vi "inclinometerSerialTest.vi"() -> ()   [LabVIEW 2016]
uses:
  <vilib>/Instr/_visa.llb/VISA Configure Serial Port (Instr).vi
  Common_RT_Modbus/CRC/CRC.lvclass
panel:
  out "result":i32
  out "Response":u8[](array[numeric])
  in  "Command":u8[](array[numeric])=[127, 0, 0, 0, 0, 0, 0, 0, 2, 206, 21] format="%02x"
  in  "SendMany":bool
  out "Time (us)":u32
  in  "Send":bool
  in  "Stop":bool
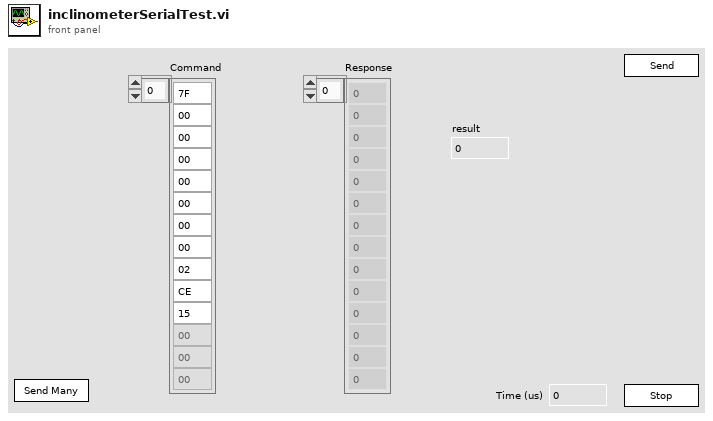
[diagram p1: front panel]
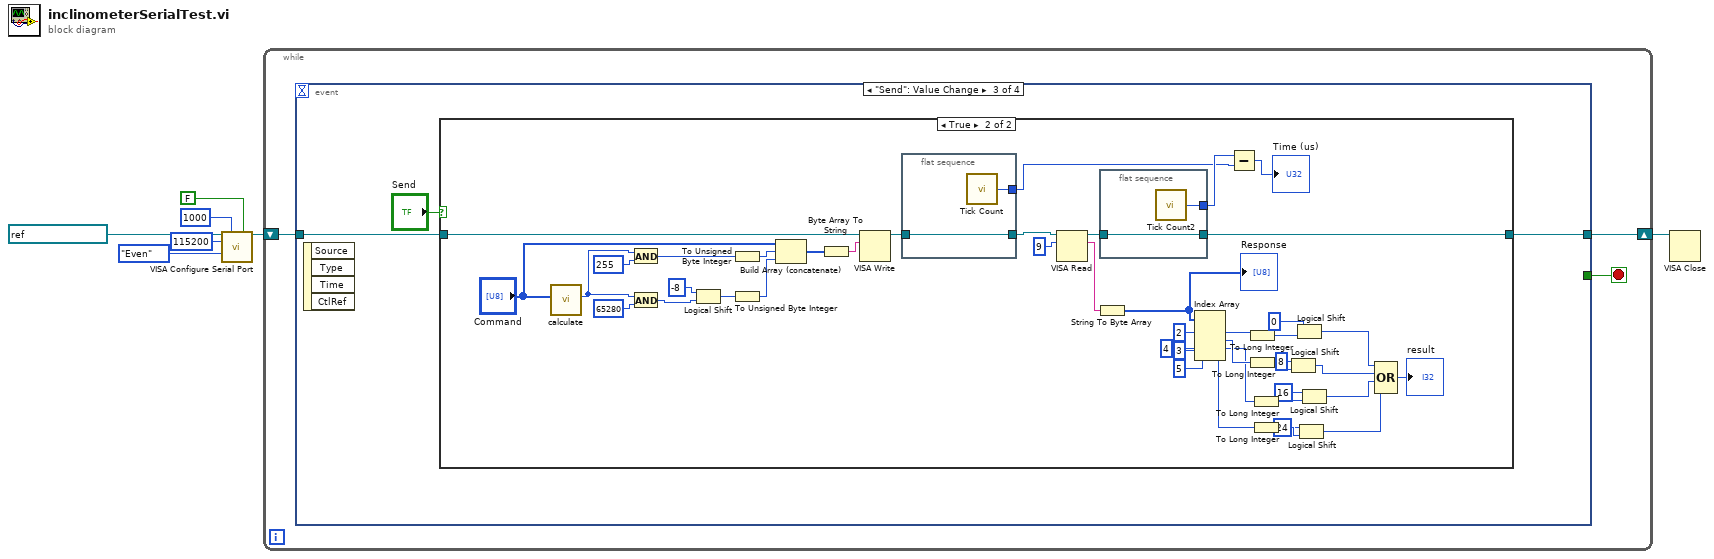
[diagram p0: block diagram]
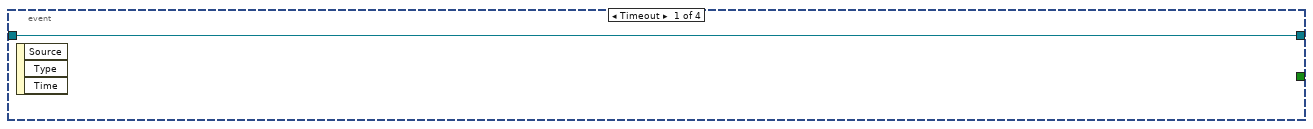
[diagram p2: hidden frame]
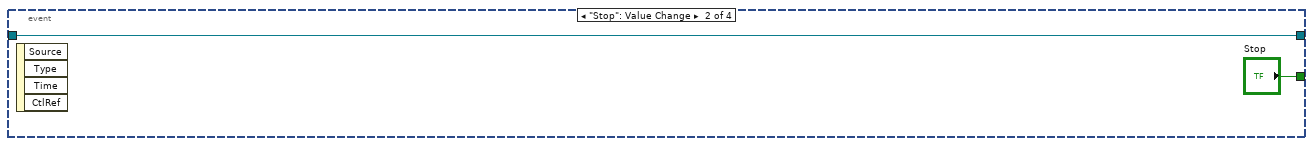
[diagram p3: hidden frame]
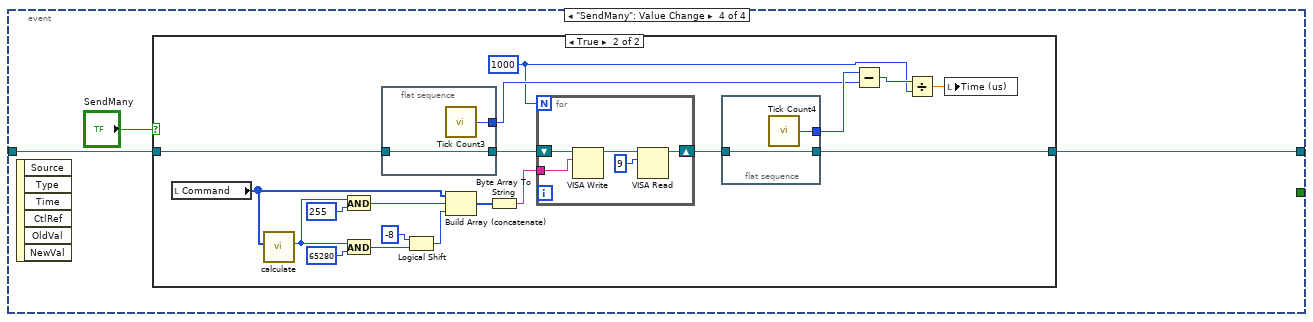
[diagram p5: hidden frame]
diagram:
  n1 = call-poly "VISA Configure Serial Port"("VISA resource name"=refnum<visa-resource-name> "ASRL1::INSTR", "timeout (10sec)"=u32 1000, "Enable Termination\nChar (T)"=FALSE ("Enable Termination\nChar (T)"), "baud rate (9600)"=u32 115200, "parity (0:none)"=enum16{"None", "Odd", "Even", "Mark", "Space"}."Even") -> ("VISA resource name out"=w3:refnum<visa-resource-name>)  [unwired: 9 in, 1 out]
  n2 = while {
    shift-right: [w9] -> w5
    shift-left: w3 -> [w10]
    stop <- w8 stop-if-true
    n3 = event shown="[2] \"Send\": Value Change" {
      selector: _ -> [_ _ _ _]
      dyn-events: _ -> [_ _ _ _]
      timeout: _ -> [_ _ _ _]
      tunnel: w10 -> [w11 w13 w15 w67]
      tunnel: [w11 w13 w14 w66] -> w9
      tunnel: [_ "Stop" _ _] -> w8
      event Timeout {
        n4 = event-data() -> ()  [unwired: 1 in, 3 out]
      }
      event "Stop": Value Change {
        n5 = event-data() -> ()  [unwired: 1 in, 4 out]
      }
      event "Send": Value Change {
        n6 = event-data() -> ()  [unwired: 1 in, 4 out]
        n7 = case shown="True" "Send" {
          tunnel: w15 -> [w17 w61]
          tunnel: [w17 w56] -> w14
          frame False {
          }
          frame True {
            n8 = call "calculate.vi"("Data"="Command") -> ("CRC"=w49:u16)  [unwired: 8 in, 2 out]
            n9 = And(x=w49, y=u16 255) -> (x .and. y?=w42:u16)
            n10 = And(x=w49, y=u16 65280) -> (x .and. y?=w46:u16)
            n11 = Logical Shift(y=i16 -8, x=w46) -> (x << y=w43:u16)
            n12 = To Unsigned Byte Integer(number=w42) -> (unsigned 8bit integer=w41:u8)
            n13 = To Unsigned Byte Integer(number=w43) -> (unsigned 8bit integer=w40:u8)
            n14 = Build Array (concatenate)("Command", w41, w40) -> (w44:u8[])
            n15 = Byte Array To String(unsigned byte array=w44) -> (string=w52:string)
            n16 = VISA Write(VISA resource name=w61, write buffer=w52) -> (VISA resource name out=w59:refnum<visa-resource-name>)  [unwired: 1 in, 2 out]
            n17 = flat-sequence {
              tunnel: w59 -> [w65]
              tunnel: [w65] -> w58
              tunnel: [w64] -> w54
              frame #0 {
                n18 = call "Tick Count"() -> ("Tick Count(uSec)"=w64:u32)
              }
            }
            n19 = VISA Read(VISA resource name=w58, byte count=u32 9) -> (VISA resource name out=w57:refnum<visa-resource-name>, read buffer=w51:string)  [unwired: 1 in, 2 out]
            n20 = String To Byte Array(string=w51) -> (unsigned byte array=w39:u8[])
            "Response" <- w39
            n21 = flat-sequence {
              tunnel: w57 -> [w63]
              tunnel: [w63] -> w56
              tunnel: [w62] -> w55
              frame #0 {
                n22 = call "Tick Count2"() -> ("Tick Count(uSec)"=w62:u32)
              }
            }
            n23 = Index Array(array=w39, index #1=2 ("index"), index #2=3 ("index"), index #3=4 ("index"), index #4=5 ("index")) -> (element #1=w33:u8, element #2=w32:u8, element #3=w27:u8, element #4=w23:u8)
            n24 = Subtract(x=w55, y=w54) -> (x-y=→"Time (us)":u32)
            n25 = To Long Integer(number=w33) -> (32bit integer=w34:i32)
            n26 = To Long Integer(number=w32) -> (32bit integer=w31:i32)
            n27 = To Long Integer(number=w27) -> (32bit integer=w28:i32)
            n28 = To Long Integer(number=w23) -> (32bit integer=w25:i32)
            n29 = Logical Shift(y=i16 8, x=w31) -> (x << y=w21:i32)
            n30 = Logical Shift(y=i16 0, x=w34) -> (x << y=w22:i32)
            n31 = Logical Shift(y=i16 24, x=w25) -> (x << y=w19:i32)
            n32 = Logical Shift(y=i16 16, x=w28) -> (x << y=w20:i32)
            n33 = Compound Arithmetic op=OR(w22, w21, w20, w19) -> (→"result":i32)
          }
        }
      }
      event "SendMany": Value Change {
        n34 = event-data() -> ()  [unwired: 1 in, 6 out]
        n35 = case shown="True" "SendMany" {
          tunnel: w67 -> [w69 w88]
          tunnel: [w69 w85] -> w66
          frame False {
          }
          frame True {
            w81 = 1000
            n36 = local read "Command"() -> (w79:u8[])
            n37 = call "calculate.vi"("Data"=w79) -> ("CRC"=w73:u16)  [unwired: 8 in, 2 out]
            n38 = And(x=w73, y=u16 255) -> (x .and. y?=w78:u16)
            n39 = And(x=w73, y=u16 65280) -> (x .and. y?=w74:u16)
            n40 = flat-sequence {
              tunnel: w88 -> [w92]
              tunnel: [w92] -> w87
              tunnel: [w91] -> w83
              frame #0 {
                n41 = call "Tick Count3"() -> ("Tick Count(uSec)"=w91:u32)
              }
            }
            n42 = Logical Shift(y=i16 -8, x=w74) -> (x << y=w77:u16)
            n43 = Build Array (concatenate)(w79, w78, w77) -> (w76:u16[])
            n44 = Byte Array To String(unsigned byte array=w76) -> (string=w71:string)
            n45 = for {
              N: w81 -> [_]
              shift-right: [w94] -> w86
              shift-left: w87 -> [w97]
              tunnel: w71 -> [w93]
              n46 = VISA Write(VISA resource name=w97, write buffer=w93) -> (VISA resource name out=w95:refnum<visa-resource-name>)  [unwired: 1 in, 2 out]
              n47 = VISA Read(VISA resource name=w95, byte count=u32 9) -> (VISA resource name out=w94:refnum<visa-resource-name>)  [unwired: 1 in, 3 out]
            }
            n48 = flat-sequence {
              tunnel: w86 -> [w90]
              tunnel: [w90] -> w85
              tunnel: [w89] -> w84
              frame #0 {
                n49 = call "Tick Count4"() -> ("Tick Count(uSec)"=w89:u32)
              }
            }
            n50 = Subtract(x=w84, y=w83) -> (x-y=w82:u32)
            n51 = Divide(x=w82, y=w81) -> (x/y=w80:dbl)
            n52 = local write "Time (us)"(w80) -> ()
          }
        }
      }
    }
  }
  n53 = VISA Close(VISA resource name=w5) -> ()  [unwired: 1 in, 1 out]
